vi "Process Input.vi"(5 "Reset":i32, 6 "Mode":i32, 7 "Switch Control":i32, 8 "error in":errorcluster, 9 "Voltage Setpoint":dbl, 10 "Current Setpoint":dbl, 11 "RMXPowerSupply in":refnum<class "RMXPowerSupply.lvclass">) -> (0 "error out":errorcluster, 3 "RMXPowerSupply out":refnum<class "RMXPowerSupply.lvclass">)   [LabVIEW 2023]
uses:
  Support/Class/RMXPowerSupply.lvclass
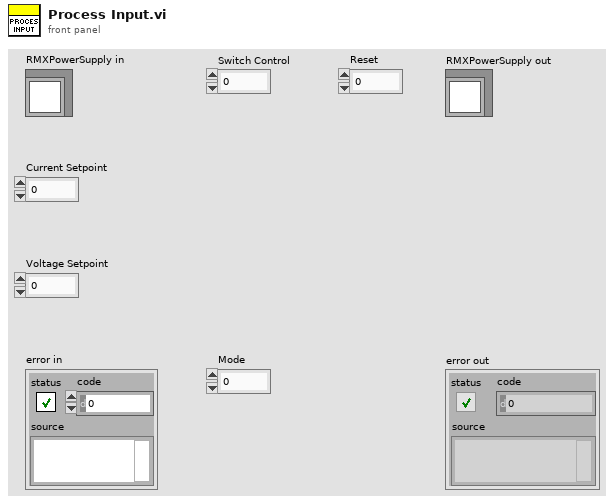
[diagram p1: front panel]
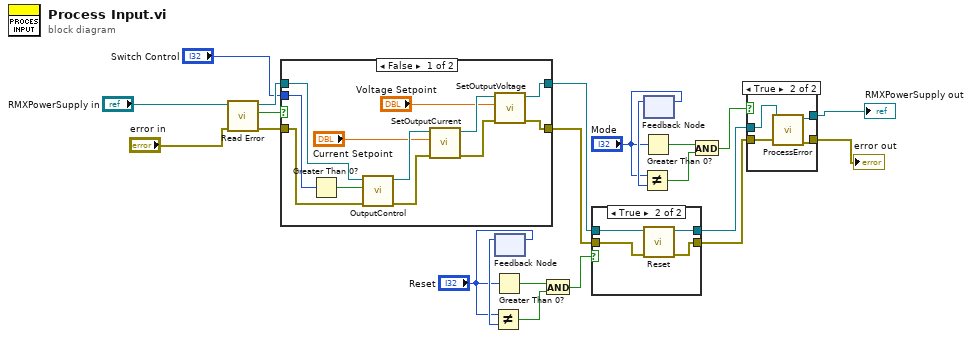
[diagram p0: block diagram]
diagram:
  n1 = call-dynamic "Read Error.vi"("error in (no error)"="error in", "RMXPowerSupply in"="RMXPowerSupply in") -> ("error out"=w21:errorcluster, "Error"=w19:bool, "RMXPowerSupply out"=w20:refnum<class "RMXPowerSupply.lvclass">)  [unwired: 7 in]
  n2 = case shown="False" w19 {
    tunnel: w20 -> [w34 w35]
    tunnel: w21 -> [w27 w36]
    tunnel: [w31 w35] -> w22
    tunnel: [w30 w36] -> w6
    tunnel: "Switch Control" -> [w28 _]
    frame False {
      n3 = Greater Than 0?(x=w28) -> (x > 0?=w29:bool)
      n4 = call-dynamic "OutputControl.vi"("error in (no error)"=w27, "On"=w29, "RMXPowerSupply in"=w34) -> ("error out"=w25:errorcluster, "RMXPowerSupply out"=w33:refnum<class "RMXPowerSupply.lvclass">)  [unwired: 7 in]
      n5 = call-dynamic "SetOutputCurrent.vi"("error in (no error)"=w25, "Current"="Current Setpoint", "RMXPowerSupply in"=w33) -> ("error out"=w23:errorcluster, "RMXPowerSupply out"=w32:refnum<class "RMXPowerSupply.lvclass">)  [unwired: 7 in]
      n6 = call-dynamic "SetOutputVoltage.vi"("error in (no error)"=w23, "Voltage"="Voltage Setpoint", "RMXPowerSupply in"=w32) -> ("error out"=w30:errorcluster, "RMXPowerSupply out"=w31:refnum<class "RMXPowerSupply.lvclass">)  [unwired: 7 in]
    }
    frame True {
    }
  }
  n7 = Greater Than 0?(x="Reset") -> (x > 0?=w15:bool)
  n8 = feedback #1() -> (w16:i32)  [unwired: 1 in]
  n9 = Not Equal?(x="Reset", y=w16) -> (x != y?=w17:bool)
  n10 = feedback-in #1("Reset") -> ()
  n11 = And(x=w15, y=w17) -> (x .and. y?=w14:bool)
  n12 = case shown="True" w14 {
    tunnel: w22 -> [w38 w42]
    tunnel: [w38 w41] -> w18
    tunnel: w6 -> [w37 w40]
    tunnel: [w37 w39] -> w4
    frame False {
    }
    frame True {
      n13 = call-dynamic "Reset.vi"("error in (no error)"=w40, "RMXPowerSupply in"=w42) -> ("error out"=w39:errorcluster, "RMXPowerSupply out"=w41:refnum<class "RMXPowerSupply.lvclass">)  [unwired: 8 in]
    }
  }
  n14 = Greater Than 0?(x="Mode") -> (x > 0?=w11:bool)
  n15 = feedback #2() -> (w12:i32)  [unwired: 1 in]
  n16 = Not Equal?(x="Mode", y=w12) -> (x != y?=w13:bool)
  n17 = feedback-in #2("Mode") -> ()
  n18 = And(x=w11, y=w13) -> (x .and. y?=w10:bool)
  n19 = case shown="True" w10 {
    tunnel: w4 -> [w44 w45]
    tunnel: [w44 w46] -> w2
    tunnel: [w43 w47] -> w3
    tunnel: w18 -> [w43 w48]
    frame False {
    }
    frame True {
      n20 = call "ProcessError.vi"("error in (no error)"=w45, "RMXPowerSupply in"=w48) -> ("error out"=w46:errorcluster, "RMXPowerSupply out"=w47:refnum<class "RMXPowerSupply.lvclass">)  [unwired: 8 in]
    }
  }
  "RMXPowerSupply out" <- w3
  "error out" <- w2
